vi "Hide Unit ID.vi"(8 "error in (no error)":errorcluster, 10 "Ctrl Ref":refnum<vi>, 11 "Item Ref in":T1 format="%.0x") -> (0 "error out":errorcluster, 3 "Item Ref out":T1 format="%.0x")   [LabVIEW 2021, in "Modbus Master System Explorer.lvlib"]
uses:
  Modbus Master System Explorer.lvlib
  <vilib>/NI VeriStand/Custom Device API/Custom Device Item Ref.ctl
  Shared/Controls/Interface Type.ctl
  Shared/Constants.vi
  <vilib>/NI VeriStand/Custom Device API/Get Item Property (U16).vi
  <vilib>/NI VeriStand/Custom Device API/Custom Device API.lvlib
  Shared/Modbus Master Shared.lvlib
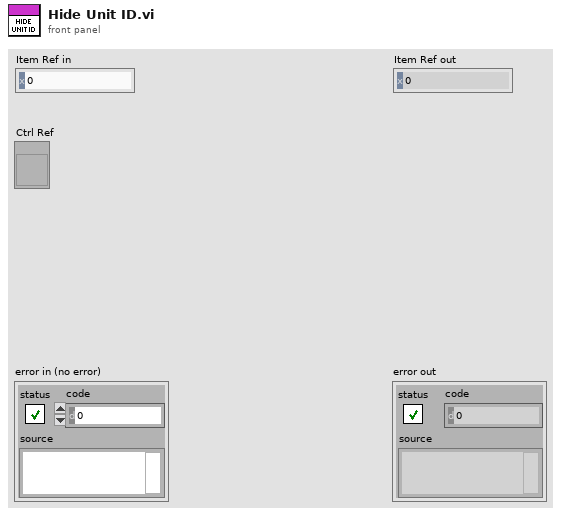
[diagram p1: front panel]
types:
  T1 = typedef "Custom Device API.lvlib/Custom Device Item Ref.ctl" = u64
  T2 = typedef "Modbus Master Shared.lvlib/Interface Type.ctl" = enum16{"TCP Master", "Serial Master", "TCP Slave", "Serial Slave"}
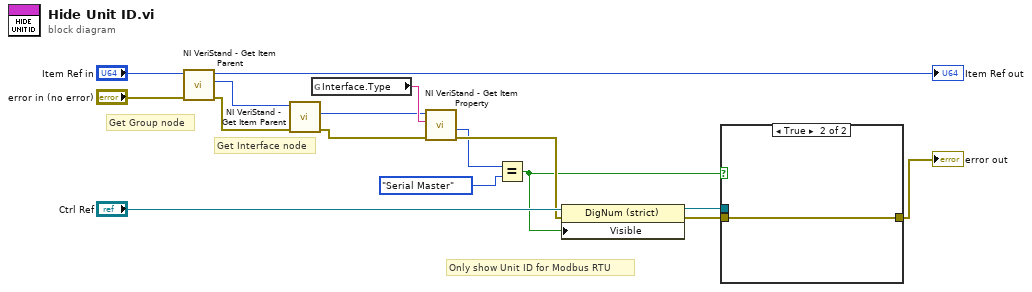
[diagram p0: block diagram]
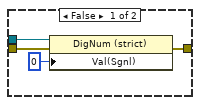
[diagram p2: hidden frame]
diagram:
  # "Only show Unit ID for Modbus RTU"
  # "Get Interface node"
  # "Get Group node"
  n1 = call <vilib>:"NI VeriStand - Get Item Parent.vi"("error in (no error)"="error in (no error)", "Item Ref in"="Item Ref in") -> ("error out"=w12:errorcluster, "Parent Ref"=w14:T1, "Item Ref out"=→"Item Ref out":T1)  [unwired: 6 in, 1 out]
  n2 = call <vilib>:"NI VeriStand - Get Item Parent.vi"("error in (no error)"=w12, "Item Ref in"=w14) -> ("error out"=w9:errorcluster, "Parent Ref"=w10:T1)  [unwired: 6 in, 2 out]
  n3 = global read "Constants.vi" "Interface.Type"() -> (w11:string)
  n4 = call-poly <vilib>:"NI VeriStand - Get Item Property.vi"("error in (no error)"=w9, "Property Name"=w11, "Item Ref in"=w10) -> ("error out"=w7:errorcluster, "Value"=w6:u16)  [unwired: 5 in, 2 out]
  n5 = Equal?(x=w6, y=Interface_Type."Serial Master" ("Interface Type")) -> (x = y?=w2:bool)
  n6 = property class="DigNum (strict)"(reference="Ctrl Ref", error in=w7, "Visible"=w2) -> (reference out=w4:refnum<vi>, error out=w3:errorcluster)
  n7 = case shown="True" w2 {
    tunnel: w4 -> [w20 _]
    tunnel: w3 -> [w19 w21]
    tunnel: [w17 w21] -> w1
    frame False {
      n8 = property class="DigNum (strict)"(reference=w20, error in=w19, "Val(Sgnl)"=u8 0 ("Value (Signaling)")) -> (error out=w17:errorcluster)  [unwired: 1 out]
    }
    frame True {
    }
  }
  "error out" <- w1
